vi "GoToSkill_v2_Init.vi"(0 "object in":refnum<class "GoToSkill_v2.lvclass">, 5 "error in (no error)":errorcluster) -> (14 "object out":refnum<class "GoToSkill_v2.lvclass">, 19 "error out":errorcluster)   [LabVIEW 2023, in "GoToSkill_v2.lvclass"]
uses:
  GoToSkill_v2.lvclass
  C:/Users/ebert/Documents/codes/SSL/repo/SSL_AI/NewSTP/NewSkills/Skill_v2_class/Skill_v2.lvclass
  GoToSkill_v2.lvclass/GoToSkill_v2.ctl
  NewSTP/NewSkills/Skill_v2_class/Skill_v2.lvclass
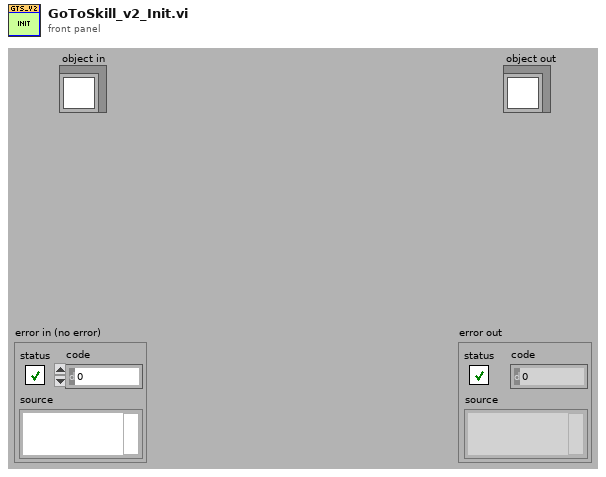
[diagram p1: front panel]
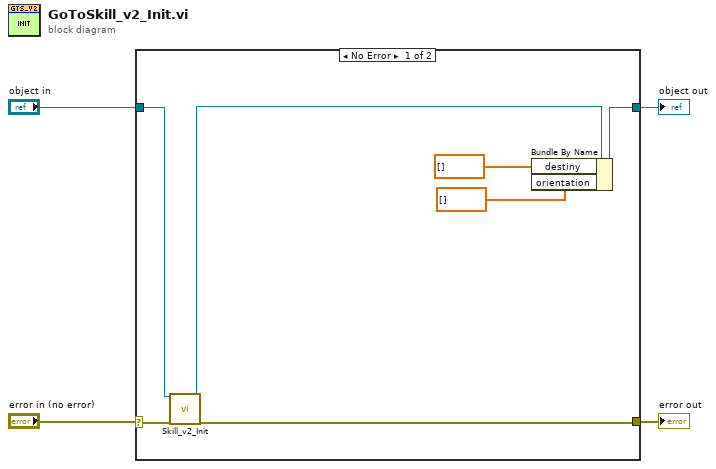
[diagram p0: block diagram]
diagram:
  n1 = case shown="No Error" "error in (no error)" {
    selector: "error in (no error)" -> [w8 w12]
    tunnel: [w11 w13] -> w4
    tunnel: "object in" -> [w10 w13]
    tunnel: [w7 w12] -> w1
    frame No Error {
      n2 = call "Skill_v2_Init.vi"("object in"=w10, "error in (no error)"=w8) -> ("object out"=w9:refnum<class "GoToSkill_v2.lvclass">, "error out"=w7:errorcluster)  [unwired: 16 in]
      n3 = Bundle By Name(cluster=w9, "destiny"=dbl[] [], "orientation"=dbl[] []) -> (w11:refnum<class "GoToSkill_v2.lvclass">)
    }
    frame Error {
    }
  }
  "object out" <- w4
  "error out" <- w1
